vi "Emergency Stop all Instruments.vi"(8 "Error In":errorcluster, 11 "reference in":refnum<class "Measure and Stimulus Subsystems.lvclass">) -> (0 "Error Out":errorcluster, 3 "reference out":refnum<class "Measure and Stimulus Subsystems.lvclass">)   [LabVIEW 2023, in "HAL GOOP4.lvlib" / "Measure and Stimulus Subsystems.lvclass"]
uses:
  Measure and Stimulus Subsystems.lvclass
  Measure and Stimulus Subsystems.lvclass/Measure and Stimulus Subsystems.ctl
  Instrument/Instrument.lvclass
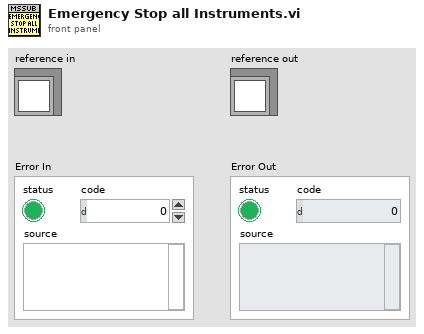
[diagram p1: front panel]
types:
  T1 = typedef "HAL GOOP4.lvlib/Measure and Stimulus Subsystems.lvclass/ObjectAttributes.ctl" = cluster{"Virt Instr":map{string, refnum<class "Virt Instr Base.lvclass">}, "Phys Instr":map{string, cluster{"Instrument":refnum<class "Instrument.lvclass">, "Ref Count":u8}}}
  T2 = map{string, cluster{"Instrument":refnum<class "Instrument.lvclass">, "Ref Count":u8}}
  T3 = cluster{"Instrument":refnum<class "Instrument.lvclass">, "Ref Count":u8}
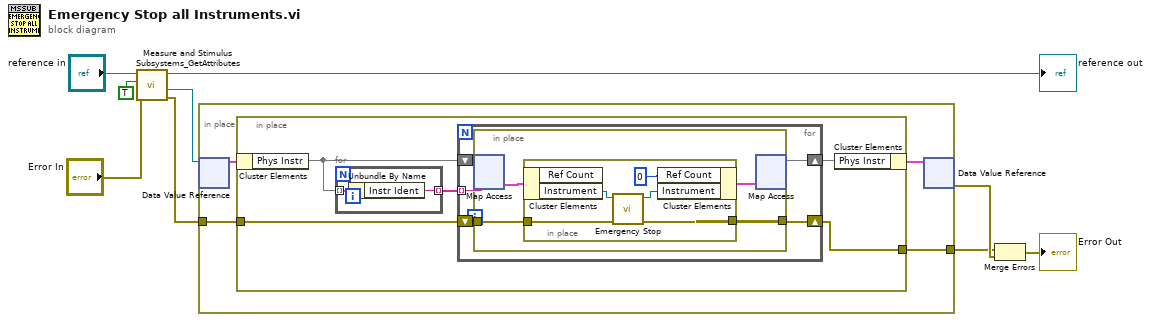
[diagram p0: block diagram]
diagram:
  n1 = call "Measure and Stimulus Subsystems_GetAttributes.vi"("Error In"="Error In", "OnlyGetDvrReference(False)"=TRUE, "reference in"="reference in") -> ("Error Out"=w2:errorcluster, "DataRef"=w3:refnum<data-value>, "reference out"=→"reference out":refnum<class "Measure and Stimulus Subsystems.lvclass">)  [unwired: 5 in, 1 out]
  n2 = in-place {
    in-place-border: w2 -> [w11]
    in-place-border: [w10] -> w1
    n3 = in-place-dvr #1(w3) -> (w13:T1)  [unwired: 1 out]
    n4 = in-place {
      in-place-border: w11 -> [w18]
      in-place-border: [w17] -> w10
      n5 = in-place-cluster #2(w13) -> ("Phys Instr"=w16:T2)
      n6 = for {
        tunnel: w16 -> [w20] mode=indexing
        tunnel: [w19] -> w15 mode=indexing
        n7 = Unbundle By Name(w20) -> ("Instr Ident"=w19:string)
      }
      n8 = for {
        shift-right: [w25] -> w17
        shift-left: w18 -> [w24]
        shift-right: [w21] -> w14
        shift-left: w16 -> [w22]
        tunnel: w15 -> [w23] mode=indexing
        n9 = in-place {
          in-place-border: [w29] -> w25
          in-place-border: w24 -> [w27]
          n10 = in-place-map #3(w22, w23) -> (w28:T3)  [unwired: 1 in, 1 out]
          n11 = in-place {
            in-place-border: [w34] -> w29
            in-place-border: w27 -> [w30]
            n12 = in-place-cluster #4(w28) -> ("Instrument"=w33:refnum<class "Instrument.lvclass">)  [unwired: 1 out]
            n13 = call "Emergency Stop.vi"("error in (no error)"=w30, "reference in"=w33) -> ("error out"=w34:errorcluster, "reference out"=w32:refnum<class "Instrument.lvclass">)  [unwired: 8 in]
            n14 = in-place-cluster #4("Ref Count"=u8 0, "Instrument"=w32) -> (w26:T3)
          }
          n15 = in-place-map #3(w26) -> (w21:T2)  [unwired: 1 in, 2 out]
        }
      }
      n16 = in-place-cluster #2("Phys Instr"=w14) -> (w12:T1)
    }
    n17 = in-place-dvr #1(w12) -> (w5:errorcluster)  [unwired: 1 out]
  }
  n18 = Merge Errors(w1, w5) -> (→"Error Out":errorcluster)
